vi "SubVI.vi"(9 "ht":dbl, 10 "uout":dbl min=0.0 max=1.0 step=0.05, 11 "uin":dbl min=0.0 max=1.0 step=0.05) -> (3 "Tank":dbl(slide) scale=0.0..10.0)   [LabVIEW 2022 SP3]
uses:
  <vilib>/express/express arith-compare/Formula/XNode/ExpressFormulaBlockNode.xnode
panel:
  in  "kout":dbl
  in  "kin":dbl
  in  "dt":dbl
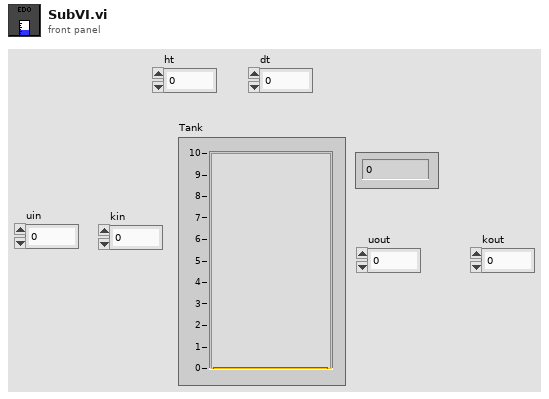
[diagram p1: front panel]
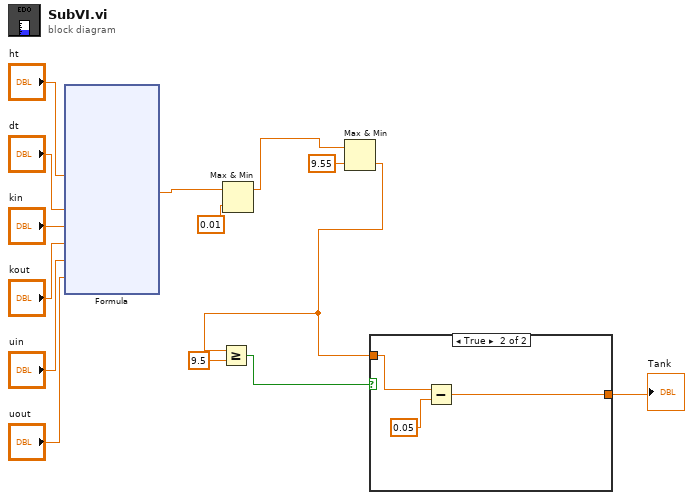
[diagram p0: block diagram]
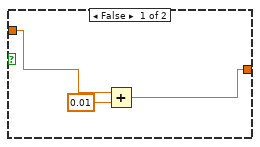
[diagram p2: hidden frame]
diagram:
  n1 = xnode "Formula"("ht"="ht", "dt"="dt", "kin"="kin", "kout"="kout", "uin"="uin", "uout"="uout") -> ("Result"=w7:dbl)  [unwired: 1 in, 1 out]
  n2 = Max & Min(x=w7, y=0.01) -> (max(x,y)=w8:dbl)  [unwired: 1 out]
  n3 = Max & Min(x=w8, y=9.55) -> (min(x,y)=w2:dbl)  [unwired: 1 out]
  n4 = Greater Or Equal?(x=w2, y=9.5) -> (x >= y?=w3:bool)
  n5 = case shown="True" w3 {
    tunnel: w2 -> [w17 w20]
    tunnel: [w16 w18] -> w1
    frame False {
      n6 = Add(x=w17, y=0.01) -> (x+y=w16:dbl)
    }
    frame True {
      n7 = Subtract(x=w20, y=0.05) -> (x-y=w18:dbl)
    }
  }
  "Tank" <- w1
